vi "lumencor_off.vi"   [LabVIEW 2011]
uses:
  <vilib>/DAQmx/write.llb/DAQmx Write (Analog 1D DBL NChan 1Samp).vi
  <vilib>/DAQmx/miscellaneous.llb/DAQmx Fill In Error Info.vi
types:
  T1 = enum32{"Invalid", "Standard", "Closed", "Hidden", "Minimized", "Maximized"}
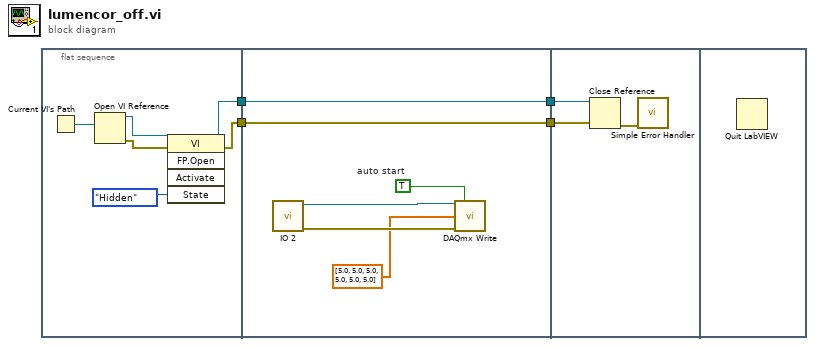
[diagram p0: block diagram]
diagram:
  n1 = flat-sequence {
    tunnel: [w6] -> w3
    tunnel: [w5] -> w1
    tunnel: [w12] -> w4
    tunnel: w3 -> [w12]
    tunnel: [w11] -> w2
    tunnel: w1 -> [w11]
    tunnel: w4 -> [w18]
    tunnel: w2 -> [w17]
    frame #0 {
      n2 = Current VI's Path() -> (path=w10:path)
      n3 = Open VI Reference(vi path=w10) -> (vi reference=w9:refnum<vi>, error out=w8:errorcluster)  [unwired: 5 in]
      n4 = invoke class="VI" method="FP.Open"(reference=w9, error in=w8, "State"=T1."Hidden") -> (reference out=w5:refnum<vi>, error out=w6:errorcluster)  [unwired: 2 in, 3 out]
    }
    frame #1 {
      w16 = TRUE  # auto start
      n5 = call "IO 2.vi"() -> ("error out"=w14:errorcluster, "task out"=w15:refnum<k21>)  [unwired: 10 in]
      n6 = call-poly <vilib>:"DAQmx Write.vi"("task/channels in"=w15, "auto start"=w16, "data"=dbl[] [5.0, 5.0, 5.0, 5.0, 5.0, 5.0], "error in"=w14) -> ()  [unwired: 12 out]
    }
    frame #2 {
      n7 = Close Reference(reference=w17, error in (no error)=w18) -> (error out=w19:errorcluster)
      n8 = call <vilib>:"Simple Error Handler.vi"("error in (no error)"=w19) -> ()  [unwired: 4 in, 5 out]
    }
    frame #3 {
      n9 = Quit LabVIEW() -> ()  [unwired: 1 in]
    }
  }
